vi "Cast Connection Callback VI.vi"(11 "VI":refnum<vi>) -> (2 "error out":errorcluster, 3 "Casted Ref":refnum<vi>)   [LabVIEW 2020, in "Stream-Simple-Msg.lvlib" / "Manager.lvclass"]
uses:
  Manager.lvclass
  Endpoint/Endpoint.lvclass
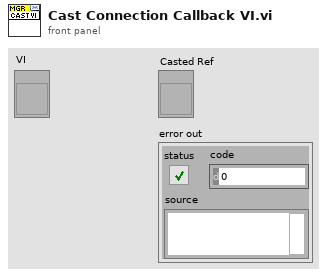
[diagram p1: front panel]
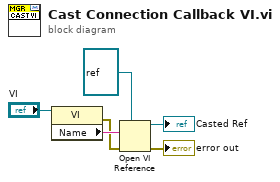
[diagram p0: block diagram]
diagram:
  n1 = property class="VI"(reference="VI") -> (error out=w4:errorcluster, "Name"=w6:string)  [unwired: 1 in, 1 out]
  n2 = Open VI Reference(type specifier VI Refnum (for type only)=refnum<vi> refnum, vi path=w6, error in (no error)=w4) -> (vi reference=→"Casted Ref":refnum<vi>, error out=→"error out":errorcluster)  [unwired: 3 in]
